vi "LSMcontroller_v64_updatedwaveformhandling.vi"() -> ()   [LabVIEW 2015] (continued)
                                "frames recorded" <- w3245
                                n916 = Greater?(x=w3258, y=w3260) -> (0:w3259:bool)
                                n917 = Quotient & Remainder(x=w3246, y=w3245) -> (floor(x/y)=w3247:i32)  [unwired: 1 out]
                                n918 = Transpose 2D Array(2D array=w3255) -> (transposed array=w3249:u16[][])
                                n919 = Transpose 2D Array(2D array=w3253) -> (transposed array=w3254:sgl[][])
                                n920 = And(x=w3259, y=w3248) -> (x .and. y?=w3261:bool)
                                n921 = local write "img_CH2"(w3254) -> ()
                                n922 = local write "photons/frame"(w3247) -> ()
                                n923 = Array Max & Min(array=w3249) -> (max value=w3250:u16)  [unwired: 3 out]
                                n924 = To Single Precision Float(number=w3249) -> (single precision float=w3252:sgl[][])
                                n925 = case shown="True" w3261 {
                                tunnel: w3260 -> [_ w3265]
                                frame False {
                                }
                                frame True {
                                n926 = Quotient & Remainder(x=w3265, y=u32 2 ("min phot")) -> (floor(x/y)=w3264:u32)  [unwired: 1 out]
                                n927 = Max & Min(x=w3264, y=u32 5) -> (max(x,y)=w3263:u32)  [unwired: 1 out]
                                n928 = local write "min phot"(w3263) -> ()
                                }
                                }
                                n929 = To Double Precision Float(number=w3250) -> (double precision float=w3251:dbl)
                                n930 = local write "img_CH1"(w3252) -> ()
                                n931 = property on="img_CH1" class="IntGraph (strict)"("ZScale.Maximum"=w3251) -> ()  [unwired: 2 in, 2 out]
                                }
                                }
                                }
                                frame #4 {
                                w3269 = u16 1 items=["Stream to disk", "Post process", "real time process"] ("Ring")
                                n932 = local read "T3R Data processing"() -> (w3268:u16)
                                n933 = Equal?(x=w3268, y=w3269) -> (x = y?=w3267:bool)
                                n934 = case shown="False" w3267 {
                                frame False {
                                # "intensity"
                                n935 = local read "Current Average"() -> (w3274:sgl)
                                n936 = local read "image2list"() -> (w3270:u16)
                                n937 = local read "image1list"() -> (w3271:u16)
                                n938 = call "dattoimage.vi"("image2list"=w3270, "Current Average"=w3274, "image1list"=w3271) -> ("image 1 array out"=w3273:sgl[][])  [unwired: 1 out]
                                n939 = Transpose 2D Array(2D array=w3273) -> (transposed array=w3272:sgl[][])
                                n940 = local write "img_CH2"(w3272) -> ()
                                }
                                frame True {
                                }
                                }
                                }
                                }
                              }
                              frame Enabled {
                              }
                            }
                          }
                        }
                        n941 = local write "64bit disabled"(TRUE ("64bit disabled")) -> ()
                      }
                      frame #9 {
                        n942 = call "2pparameters.vi"("command"="get") -> ("params out"=w3277:T10)  [unwired: 1 in]
                        n943 = Unbundle By Name(w3277) -> ("auto OD"=w3276:bool)
                        n944 = case shown="True" w3276 {
                          frame False {
                          }
                          frame True {
                            n945 = call "configuration.vi"("command"="get") -> ("config out"=w3280:T11)  [unwired: 2 in, 1 out]
                            n946 = call "2pparameters.vi"("command"="get") -> ("params out"=w3283:T10)  [unwired: 1 in]
                            n947 = Unbundle By Name(w3280) -> ("image OD"=w3278:u16)
                            n948 = Unbundle By Name(w3283) -> ("ODfilt"=w3279:u16)
                            n949 = call "filterwheelcontrol_nothorlabslib.vi"("Current OD filt"=w3278, "New ODfilt"=w3279) -> ()  [unwired: 1 in]
                          }
                        }
                        n950 = call "reset AO_DO_v3.vi"() -> ()  [unwired: 12 in]
                      }
                      frame #10 {
                        n951 = stacked-sequence {
                          tunnel: w3297 -> [w3300 _ _ _ _ _]
                          tunnel: w3296 -> [w3299 _ _ _ _ _]
                          tunnel: w3295 -> [w3298 _ _ _ _ _]
                          tunnel: w3294 -> [_ w3349 _ _ _ _]
                          tunnel: w3293 -> [_ w3348 w3403 w3500 _ _]
                          tunnel: w3292 -> [_ w3347 w3402 w3499 _ _]
                          tunnel: w3291 -> [_ _ w3401 _ _ _]
                          tunnel: w3290 -> [_ _ w3400 _ _ _]
                          tunnel: w3289 -> [_ _ _ w3498 _ _]
                          tunnel: w3288 -> [_ _ _ w3497 _ _]
                          tunnel: w3287 -> [_ _ w3398 _ _ _]
                          tunnel: w3286 -> [_ _ w3397 _ _ _]
                          tunnel: w3285 -> [_ _ _ w3495 _ _]
                          tunnel: w3284 -> [_ _ _ w3494 _ _]
                          frame #0 {
                            n952 = case shown="False" w3300 {
                              tunnel: w3299 -> [_ w3322]
                              tunnel: w3298 -> [_ w3321]
                              frame True {
                                n953 = stacked-sequence {
                                seq-local: [w3301 _ _] -> [_ w3313 w3318]
                                frame #0 {
                                n954 = call "configuration.vi"("command"="get") -> ("config out"=w3307:T11)  [unwired: 2 in, 1 out]
                                n955 = Unbundle By Name(w3307) -> ("Voltage to Xgalvo"=w3304:i32)
                                n956 = call "2pparameters.vi"("command"="get") -> ("params out"=w3305:T10)  [unwired: 1 in]
                                n957 = in-place {
                                in-place-border: w3304 -> [w3312]
                                in-place-border: [w3309] -> w3301
                                n958 = in-place-cluster #9(w3305) -> ("aAO"=w3311:u32[])
                                n959 = call "remove channel from active arrayv2.vi"("line array in"=w3311, "line to remove"=w3312) -> ("line array out"=w3310:u32[], "index"=w3309:i32)  [unwired: 1 out]
                                n960 = in-place-cluster #9("aAO"=w3310) -> (w3302:T10)
                                }
                                n961 = call "2pparameters.vi"("Params in"=w3302, "command"="set") -> ()  [unwired: 1 out]
                                }
                                frame #1 {
                                n962 = call "waveformparamsv2.vi"("command"="rem AO", "index"=w3313) -> ()  [unwired: 3 in, 3 out]
                                }
                                frame #2 {
                                n963 = call "waveformsAObuffer.vi"("command"="get") -> ("AO wf out"=w3319:waveform(dbl)[])  [unwired: 1 in]
                                n964 = Delete From Array(array=w3319, length=1, index=w3318) -> (array with subset deleted=w3315:waveform(dbl)[])  [unwired: 1 out]
                                n965 = call "waveformsAObuffer.vi"("AO wf in"=w3315, "command"="set") -> ()  [unwired: 1 out]
                                }
                                }
                              }
                              frame False {
                                n966 = stacked-sequence {
                                seq-local: [w3323 _ _] -> [_ w3331 w3342]
                                tunnel: w3322 -> [_ w3330 _]
                                tunnel: w3321 -> [_ _ w3341]
                                frame #0 {
                                n967 = call "configuration.vi"("command"="get") -> ("config out"=w3328:T11)  [unwired: 2 in, 1 out]
                                n968 = Unbundle By Name(w3328) -> ("Voltage to Xgalvo"=w3324:i32)
                                n969 = call "2pparameters.vi"("command"="get") -> ("params out"=w3327:T10)  [unwired: 1 in]
                                n970 = Unbundle By Name(w3327) -> ("aAO"=w3325:u32[])
                                n971 = Search 1D Array(1D array=w3325, element=w3324) -> (index of element=w3323:i32)  [unwired: 1 in]
                                }
                                frame #1 {
                                n972 = call "waveformparamsv2.vi"("command"="get") -> ("Params out"=w3334:T14)  [unwired: 4 in, 2 out]
                                n973 = in-place {
                                in-place-border: w3331 -> [w3338]
                                in-place-border: w3330 -> [w3337]
                                n974 = in-place-cluster #10(w3334) -> ("AO parameters"=w3339:T15)
                                n975 = in-place {
                                in-place-border: w3337 -> [w3340]
                                n976 = in-place-array #11(w3339, w3338) -> ()  [unwired: 1 out]
                                n977 = in-place-array #11(w3340) -> (w3336:T15)  [unwired: 1 out]
                                }
                                n978 = in-place-cluster #10("AO parameters"=w3336) -> (w3332:T14)
                                }
                                n979 = call "waveformparamsv2.vi"("command"="set", "Params in"=w3332) -> ()  [unwired: 3 in, 3 out]
                                }
                                frame #2 {
                                n980 = call "waveformsAObuffer.vi"("command"="get") -> ("AO wf out"=w3345:waveform(dbl)[])  [unwired: 1 in]
                                n981 = Replace Array Subset(array=w3345, new element=w3341, index=w3342) -> (w3343:waveform(dbl)[])
                                n982 = call "waveformsAObuffer.vi"("AO wf in"=w3343, "command"="set") -> ()  [unwired: 1 out]
                                }
                                }
                              }
                            }
                          }
                          frame #1 {
                            n983 = case shown="True" w3349 {
                              tunnel: w3348 -> [_ w3371]
                              tunnel: w3347 -> [_ w3370]
                              frame True {
                                n984 = stacked-sequence {
                                seq-local: [w3350 _ _] -> [_ w3362 w3367]
                                frame #0 {
                                n985 = call "configuration.vi"("command"="get") -> ("config out"=w3356:T11)  [unwired: 2 in, 1 out]
                                n986 = Unbundle By Name(w3356) -> ("Voltage to Ygalvo"=w3353:i32)
                                n987 = call "2pparameters.vi"("command"="get") -> ("params out"=w3354:T10)  [unwired: 1 in]
                                n988 = in-place {
                                in-place-border: w3353 -> [w3361]
                                in-place-border: [w3358] -> w3350
                                n989 = in-place-cluster #12(w3354) -> ("aAO"=w3360:u32[])
                                n990 = call "remove channel from active arrayv2.vi"("line array in"=w3360, "line to remove"=w3361) -> ("line array out"=w3359:u32[], "index"=w3358:i32)  [unwired: 1 out]
                                n991 = in-place-cluster #12("aAO"=w3359) -> (w3351:T10)
                                }
                                n992 = call "2pparameters.vi"("Params in"=w3351, "command"="set") -> ()  [unwired: 1 out]
                                }
                                frame #1 {
                                n993 = call "waveformparamsv2.vi"("command"="rem AO", "index"=w3362) -> ()  [unwired: 3 in, 3 out]
                                }
                                frame #2 {
                                n994 = call "waveformsAObuffer.vi"("command"="get") -> ("AO wf out"=w3368:waveform(dbl)[])  [unwired: 1 in]
                                n995 = Delete From Array(array=w3368, length=1, index=w3367) -> (array with subset deleted=w3364:waveform(dbl)[])  [unwired: 1 out]
                                n996 = call "waveformsAObuffer.vi"("AO wf in"=w3364, "command"="set") -> ()  [unwired: 1 out]
                                }
                                }
                              }
                              frame False {
                                n997 = stacked-sequence {
                                seq-local: [w3372 _ _] -> [_ w3380 w3391]
                                tunnel: w3371 -> [_ w3379 _]
                                tunnel: w3370 -> [_ _ w3390]
                                frame #0 {
                                n998 = call "configuration.vi"("command"="get") -> ("config out"=w3377:T11)  [unwired: 2 in, 1 out]
                                n999 = Unbundle By Name(w3377) -> ("Voltage to Ygalvo"=w3373:i32)
                                n1000 = call "2pparameters.vi"("command"="get") -> ("params out"=w3376:T10)  [unwired: 1 in]
                                n1001 = Unbundle By Name(w3376) -> ("aAO"=w3374:u32[])
                                n1002 = Search 1D Array(1D array=w3374, element=w3373) -> (index of element=w3372:i32)  [unwired: 1 in]
                                }
                                frame #1 {
                                n1003 = call "waveformparamsv2.vi"("command"="get") -> ("Params out"=w3383:T14)  [unwired: 4 in, 2 out]
                                n1004 = in-place {
                                in-place-border: w3380 -> [w3387]
                                in-place-border: w3379 -> [w3386]
                                n1005 = in-place-cluster #13(w3383) -> ("AO parameters"=w3388:T15)
                                n1006 = in-place {
                                in-place-border: w3386 -> [w3389]
                                n1007 = in-place-array #14(w3388, w3387) -> ()  [unwired: 1 out]
                                n1008 = in-place-array #14(w3389) -> (w3385:T15)  [unwired: 1 out]
                                }
                                n1009 = in-place-cluster #13("AO parameters"=w3385) -> (w3381:T14)
                                }
                                n1010 = call "waveformparamsv2.vi"("command"="set", "Params in"=w3381) -> ()  [unwired: 3 in, 3 out]
                                }
                                frame #2 {
                                n1011 = call "waveformsAObuffer.vi"("command"="get") -> ("AO wf out"=w3394:waveform(dbl)[])  [unwired: 1 in]
                                n1012 = Replace Array Subset(array=w3394, new element=w3390, index=w3391) -> (w3392:waveform(dbl)[])
                                n1013 = call "waveformsAObuffer.vi"("AO wf in"=w3392, "command"="set") -> ()  [unwired: 1 out]
                                }
                                }
                              }
                            }
                          }
                          frame #2 {
                            n1014 = Build Array(w3398, w3397) -> (w3396:bool[])
                            n1015 = Boolean Array To Number(Boolean array=w3396) -> (number=w3399:u32)
                            n1016 = case shown="0" w3399 {
                              tunnel: w3403 -> [_ _ w3446]
                              tunnel: w3402 -> [_ _ w3445]
                              tunnel: w3401 -> [_ w3425 w3443]
                              tunnel: w3400 -> [_ w3424 w3444]
                              frame 1, Default {
                                n1017 = stacked-sequence {
                                seq-local: [w3404 _ _] -> [_ w3416 w3421]
                                frame #0 {
                                n1018 = call "configuration.vi"("command"="get") -> ("config out"=w3410:T11)  [unwired: 2 in, 1 out]
                                n1019 = Unbundle By Name(w3410) -> ("2P shutter"=w3407:i32)
                                n1020 = call "2pparameters.vi"("command"="get") -> ("params out"=w3408:T10)  [unwired: 1 in]
                                n1021 = in-place {
                                in-place-border: w3407 -> [w3415]
                                in-place-border: [w3412] -> w3404
                                n1022 = in-place-cluster #15(w3408) -> ("aDO"=w3414:u32[])
                                n1023 = call "remove channel from active arrayv2.vi"("line array in"=w3414, "line to remove"=w3415) -> ("line array out"=w3413:u32[], "index"=w3412:i32)  [unwired: 1 out]
                                n1024 = in-place-cluster #15("aDO"=w3413) -> (w3405:T10)
                                }
                                n1025 = call "2pparameters.vi"("Params in"=w3405, "command"="set") -> ()  [unwired: 1 out]
                                }
                                frame #1 {
                                n1026 = call "waveformparamsv2.vi"("command"="rem DO", "index"=w3416) -> ()  [unwired: 3 in, 3 out]
                                }
                                frame #2 {
                                n1027 = call "waveformsDObuffer.vi"("command"="get") -> ("DO wf out"=w3422:digitalwaveform[])  [unwired: 1 in]
                                n1028 = Delete From Array(array=w3422, length=1, index=w3421) -> (array with subset deleted=w3418:digitalwaveform[])  [unwired: 1 out]
                                n1029 = call "waveformsDObuffer.vi"("DO wf in"=w3418, "command"="set") -> ()  [unwired: 1 out]
                                }
                                }
                              }
                              frame 2 {
                                n1030 = stacked-sequence {
                                tunnel: w3425 -> [_ w3436 _]
                                tunnel: w3424 -> [_ _ w3440]
                                frame #0 {
                                n1031 = call "configuration.vi"("command"="get") -> ("config out"=w3427:T11)  [unwired: 2 in, 1 out]
                                n1032 = call "2pparameters.vi"("command"="get") -> ("params out"=w3431:T10)  [unwired: 1 in]
                                n1033 = Unbundle By Name(w3427) -> ("2P shutter"=w3426:i32)
                                n1034 = in-place {
                                in-place-border: w3426 -> [w3435]
                                n1035 = in-place-cluster #16(w3431) -> ("aDO"=w3434:u32[])
                                n1036 = call "add channel to active arrayv2.vi"("line array in"=w3434, "line to add"=w3435) -> ("line array out"=w3433:u32[])  [unwired: 2 out]
                                n1037 = in-place-cluster #16("aDO"=w3433) -> (w3429:T10)
                                }
                                n1038 = call "2pparameters.vi"("Params in"=w3429, "command"="set") -> ()  [unwired: 1 out]
                                }
                                frame #1 {
                                n1039 = call "waveformparamsv2.vi"("command"="add DO", "add DO"=w3436) -> ()  [unwired: 3 in, 3 out]
                                }
                                frame #2 {
                                n1040 = call "waveformsDObuffer.vi"("command"="get") -> ("DO wf out"=w3441:digitalwaveform[])  [unwired: 1 in]
                                n1041 = Build Array (concatenate)(w3441, w3440) -> (w3439:digitalwaveform[])
                                n1042 = call "waveformsDObuffer.vi"("DO wf in"=w3439, "command"="set") -> ()  [unwired: 1 out]
                                }
                                }
                              }
                              frame 0 {
                                n1043 = stacked-sequence {
                                seq-local: [w3447 _ _] -> [_ w3455 w3477]
                                tunnel: w3446 -> [_ _ _]
                                tunnel: w3445 -> [_ _ _]
                                tunnel: w3444 -> [_ _ w3476]
                                tunnel: w3443 -> [_ w3454 _]
                                frame #0 {
                                n1044 = call "configuration.vi"("command"="get") -> ("config out"=w3452:T11)  [unwired: 2 in, 1 out]
                                n1045 = call "2pparameters.vi"("command"="get") -> ("params out"=w3451:T10)  [unwired: 1 in]
                                n1046 = Unbundle By Name(w3452) -> ("2P shutter"=w3448:i32)
                                n1047 = Unbundle By Name(w3451) -> ("aDO"=w3449:u32[])
                                n1048 = Search 1D Array(1D array=w3449, element=w3448) -> (index of element=w3447:i32)  [unwired: 1 in]
                                }
                                frame #1 {
                                n1049 = call "2pparameters.vi"("command"="get") -> ("params out"=w3458:T10)  [unwired: 1 in]
                                n1050 = Unbundle By Name(w3458) -> ("wavdet"=w3456:bool, "autoshutter"=w3457:bool)
                                n1051 = case shown="True" w3457 {
                                tunnel: w3455 -> [_ w3462]
                                tunnel: w3456 -> [_ w3461]
                                tunnel: w3454 -> [_ w3460]
                                frame False {
                                }
                                frame True {
                                n1052 = case shown="False" w3461 {
                                tunnel: w3462 -> [w3466 _]
                                tunnel: w3460 -> [w3464 _]
                                frame False {
                                n1053 = Index Array(array=w3464, index=0) -> (element=w3463:T18)
                                n1054 = call "waveformparamsv2.vi"("command"="get") -> ("Params out"=w3469:T14)  [unwired: 4 in, 2 out]
                                n1055 = in-place {
                                in-place-border: w3466 -> [w3473]
                                in-place-border: w3463 -> [w3471]
                                n1056 = in-place-cluster #17(w3469) -> ("DO parameters"=w3474:T17)
                                n1057 = in-place {
                                in-place-border: w3471 -> [w3475]
                                n1058 = in-place-array #18(w3474, w3473) -> ()  [unwired: 1 out]
                                n1059 = in-place-array #18(w3475) -> (w3472:T17)  [unwired: 1 out]
                                }
                                n1060 = in-place-cluster #17("DO parameters"=w3472) -> (w3467:T14)
                                }
                                n1061 = call "waveformparamsv2.vi"("command"="set", "Params in"=w3467) -> ()  [unwired: 3 in, 3 out]
                                }
                                frame True {
                                }
                                }
                                }
                                }
                                }
                                frame #2 {
                                n1062 = call "2pparameters.vi"("command"="get") -> ("params out"=w3480:T10)  [unwired: 1 in]
                                n1063 = Unbundle By Name(w3480) -> ("wavdet"=w3478:bool, "autoshutter"=w3479:bool)
                                n1064 = case shown="True" w3479 {
                                tunnel: w3477 -> [_ w3484]
                                tunnel: w3478 -> [_ w3483]
                                tunnel: w3476 -> [_ w3482]
                                frame False {
                                }
                                frame True {
                                n1065 = case shown="False" w3483 {
                                tunnel: w3484 -> [w3488 _]
                                tunnel: w3482 -> [w3487 _]
                                frame False {
                                n1066 = Index Array(array=w3487, index=0) -> (element=w3485:digitalwaveform)
                                n1067 = call "waveformsDObuffer.vi"("command"="get") -> ("DO wf out"=w3490:digitalwaveform[])  [unwired: 1 in]
                                n1068 = Replace Array Subset(array=w3490, new element=w3485, index=w3488) -> (w3492:digitalwaveform[])
                                n1069 = call "waveformsDObuffer.vi"("DO wf in"=w3492, "command"="set") -> ()  [unwired: 1 out]
                                }
                                frame True {
                                }
                                }
                                }
                                }
                                }
                                }
                              }
                            }
                          }
                          frame #3 {
                            n1070 = Build Array(w3495, w3494) -> (w3496:bool[])
                            n1071 = Boolean Array To Number(Boolean array=w3496) -> (number=w3493:u32)
                            n1072 = case shown="0" w3493 {
                              tunnel: w3500 -> [_ _ w3543]
                              tunnel: w3499 -> [_ _ w3542]
                              tunnel: w3498 -> [_ w3522 w3540]
                              tunnel: w3497 -> [_ w3521 w3541]
                              frame 1, Default {
                                n1073 = stacked-sequence {
                                seq-local: [w3501 _ _] -> [_ w3513 w3518]
                                frame #0 {
                                n1074 = call "configuration.vi"("command"="get") -> ("config out"=w3507:T11)  [unwired: 2 in, 1 out]
                                n1075 = Unbundle By Name(w3507) -> ("LT timestamp"=w3504:u32)
                                n1076 = call "2pparameters.vi"("command"="get") -> ("params out"=w3505:T10)  [unwired: 1 in]
                                n1077 = in-place {
                                in-place-border: w3504 -> [w3512]
                                in-place-border: [w3509] -> w3501
                                n1078 = in-place-cluster #19(w3505) -> ("aDO"=w3511:u32[])
                                n1079 = call "remove channel from active arrayv2.vi"("line array in"=w3511, "line to remove"=w3512) -> ("line array out"=w3510:u32[], "index"=w3509:i32)  [unwired: 1 out]
                                n1080 = in-place-cluster #19("aDO"=w3510) -> (w3502:T10)
                                }
                                n1081 = call "2pparameters.vi"("Params in"=w3502, "command"="set") -> ()  [unwired: 1 out]
                                }
                                frame #1 {
                                n1082 = call "waveformparamsv2.vi"("command"="rem DO", "index"=w3513) -> ()  [unwired: 3 in, 3 out]
                                }
                                frame #2 {
                                n1083 = call "waveformsDObuffer.vi"("command"="get") -> ("DO wf out"=w3519:digitalwaveform[])  [unwired: 1 in]
                                n1084 = Delete From Array(array=w3519, length=1, index=w3518) -> (array with subset deleted=w3515:digitalwaveform[])  [unwired: 1 out]
                                n1085 = call "waveformsDObuffer.vi"("DO wf in"=w3515, "command"="set") -> ()  [unwired: 1 out]
                                }
                                }
                              }
                              frame 2 {
                                n1086 = stacked-sequence {
                                tunnel: w3522 -> [_ _ w3535]
                                tunnel: w3521 -> [_ w3533 _]
                                frame #0 {
                                n1087 = call "configuration.vi"("command"="get") -> ("config out"=w3524:T11)  [unwired: 2 in, 1 out]
                                n1088 = Unbundle By Name(w3524) -> ("LT timestamp"=w3523:u32)
                                n1089 = call "2pparameters.vi"("command"="get") -> ("params out"=w3528:T10)  [unwired: 1 in]
                                n1090 = in-place {
                                in-place-border: w3523 -> [w3532]
                                n1091 = in-place-cluster #20(w3528) -> ("aDO"=w3531:u32[])
                                n1092 = call "add channel to active arrayv2.vi"("line array in"=w3531, "line to add"=w3532) -> ("line array out"=w3530:u32[])  [unwired: 2 out]
                                n1093 = in-place-cluster #20("aDO"=w3530) -> (w3526:T10)
                                }
                                n1094 = call "2pparameters.vi"("Params in"=w3526, "command"="set") -> ()  [unwired: 1 out]
                                }
                                frame #1 {
                                n1095 = call "waveformparamsv2.vi"("command"="add DO", "add DO"=w3533) -> ()  [unwired: 3 in, 3 out]
                                }
                                frame #2 {
                                n1096 = call "waveformsDObuffer.vi"("command"="get") -> ("DO wf out"=w3538:digitalwaveform[])  [unwired: 1 in]
                                n1097 = Build Array (concatenate)(w3538, w3535) -> (w3537:digitalwaveform[])
                                n1098 = call "waveformsDObuffer.vi"("DO wf in"=w3537, "command"="set") -> ()  [unwired: 1 out]
                                }
                                }
                              }
                              frame 0 {
                                n1099 = stacked-sequence {
                                seq-local: [w3544 _ _] -> [_ w3554 w3571]
                                tunnel: w3543 -> [_ _ _]
                                tunnel: w3542 -> [_ _ _]
                                tunnel: w3541 -> [_ w3551 _]
                                tunnel: w3540 -> [_ _ w3570]
                                frame #0 {
                                n1100 = call "configuration.vi"("command"="get") -> ("config out"=w3549:T11)  [unwired: 2 in, 1 out]
                                n1101 = Unbundle By Name(w3549) -> ("LT timestamp"=w3545:u32)
                                n1102 = call "2pparameters.vi"("command"="get") -> ("params out"=w3548:T10)  [unwired: 1 in]
                                n1103 = Unbundle By Name(w3548) -> ("aDO"=w3546:u32[])
                                n1104 = Search 1D Array(1D array=w3546, element=w3545) -> (index of element=w3544:i32)  [unwired: 1 in]
                                }
                                frame #1 {
                                n1105 = local read "Measurement"() -> (w3553:T4)
                                n1106 = To Unsigned Long Integer(number=w3553) -> (unsigned 32bit integer=w3552:u32)
                                n1107 = case shown="5..7" w3552 {
                                tunnel: w3554 -> [_ w3558]
                                tunnel: w3551 -> [_ w3555]
                                frame 0..4, Default {
                                }
                                frame 5..7 {
                                n1108 = Index Array(array=w3555, index=0) -> (element=w3556:T18)
                                n1109 = call "waveformparamsv2.vi"("command"="get") -> ("Params out"=w3561:T14)  [unwired: 4 in, 2 out]
                                n1110 = in-place {
                                in-place-border: w3558 -> [w3565]
                                in-place-border: w3556 -> [w3563]
                                n1111 = in-place-cluster #21(w3561) -> ("DO parameters"=w3566:T17)
                                n1112 = in-place {
                                in-place-border: w3563 -> [w3567]
                                n1113 = in-place-array #22(w3566, w3565) -> ()  [unwired: 1 out]
                                n1114 = in-place-array #22(w3567) -> (w3564:T17)  [unwired: 1 out]
                                }
                                n1115 = in-place-cluster #21("DO parameters"=w3564) -> (w3559:T14)
                                }
                                n1116 = call "waveformparamsv2.vi"("command"="set", "Params in"=w3559) -> ()  [unwired: 3 in, 3 out]
                                }
                                }
                                }
                                frame #2 {
                                n1117 = local read "Measurement"() -> (w3569:T4)
                                n1118 = To Unsigned Long Integer(number=w3569) -> (unsigned 32bit integer=w3568:u32)
                                n1119 = case shown="5..7" w3568 {
                                tunnel: w3571 -> [_ w3575]
                                tunnel: w3570 -> [_ w3573]
                                frame 0..4, Default {
                                }
                                frame 5..7 {
                                n1120 = Index Array(array=w3573, index=0) -> (element=w3572:digitalwaveform)
                                n1121 = call "waveformsDObuffer.vi"("command"="get") -> ("DO wf out"=w3577:digitalwaveform[])  [unwired: 1 in]
                                n1122 = Replace Array Subset(array=w3577, new element=w3572, index=w3575) -> (w3579:digitalwaveform[])
                                n1123 = call "waveformsDObuffer.vi"("DO wf in"=w3579, "command"="set") -> ()  [unwired: 1 out]
                                }
                                }
                                }
                                }
                              }
                            }
                          }
                          frame #4 {
                            n1124 = call "Used AO lines.vi"() -> ("used AO names"=w3582:string[], "used AO lines"=w3580:tag[])  [unwired: 2 in]
                            n1125 = control-ref of="Analog Lines Plot"() -> (w3581:refnum<vi>)
                            n1126 = control-ref of="Digital Lines Plot"() -> (w3583:refnum<vi>)
                            n1127 = call "Used DO lines.vi"() -> ("used DO names"=w3584:string[], "used DO lines"=w3585:tag[])  [unwired: 2 in]
                            n1128 = local write "Analog Used Lines"(w3580) -> ()
                            n1129 = local write "Analog Used Names"(w3582) -> ()
                            n1130 = local write "Digital Used Lines"(w3585) -> ()
                            n1131 = local write "Digital Used Names"(w3584) -> ()
                            n1132 = call "prepDOWaveplot.vi"("DigitalGraph in"=w3583, "used DO names"=w3584) -> ()  [unwired: 1 in]
                            n1133 = call "prepAOWaveplot.vi"("WaveformGraph in"=w3581, "Analog Used Names"=w3582) -> ()  [unwired: 1 in]
                          }
                          frame #5 {
                            n1134 = local read "Meastab"() -> (w3600:enum32{"X-Y Image", "Linescan", "Timetrace"})
                            n1135 = property on="refwf" class="Ring (strict)"() -> ("RingText.Text"=w3597:string)  [unwired: 2 in, 2 out]
                            n1136 = case shown="\"Timetrace\"" w3600 {
                              tunnel: [w3602 w3603] -> w3601
                              frame "X-Y Image", Default {
                                n1137 = local read "Sampling rate"() -> (w3602:dbl)
                              }
                              frame "Timetrace" {
                                n1138 = local read "srateAODOtt"() -> (w3603:dbl)
                              }
                            }
                            n1139 = call "waveformsAObuffer.vi"("command"="get") -> ("AO wf out"=w3588:waveform(dbl)[])  [unwired: 1 in]
                            n1140 = local read "wavdet"() -> (w3598:bool)
                            n1141 = call "waveformsDObuffer.vi"("command"="get") -> ("DO wf out"=w3592:digitalwaveform[])  [unwired: 1 in]
                            n1142 = call "correctwaveformsizetemp.vi"("new sampling frequency (Hz)"=w3601, "start"=FALSE, "reference waveforms to"=w3597, "Analog waveforms in"=w3588, "stop"=TRUE, "Digital waveforms in"=w3592) -> ("analog wf out"=w3594:waveform(dbl)[], "Digital wf out"=w3596:digitalwaveform[], "measpoints"=w3599:i32)
                            n1143 = local write "Analog Lines Plot"(w3594) -> ()
                            n1144 = call "GetNumCamFramesv2.vi"("Digital Waveform Graph"=w3596) -> ("Numeric"=w3595:i32)  [unwired: 10 in]
                            n1145 = local write "Digital Lines Plot"(w3596) -> ()
                            n1146 = call "waveformsDObuffer.vi"("DO wf in"=w3596, "command"="set") -> ()  [unwired: 1 out]
                            n1147 = call "waveformsAObuffer.vi"("AO wf in"=w3594, "command"="set") -> ()  [unwired: 1 out]
                            n1148 = local write "Total Camera Frames"(w3595) -> ()
                            n1149 = case shown="True" w3598 {
                              tunnel: w3599 -> [_ w3604]
                              frame False {
                              }
                              frame True {
                                n1150 = local write "# of frames"(w3604) -> ()
                              }
                            }
                          }
                        }
                        n1151 = call "stoperaseCI.vi"() -> ()  [unwired: 12 in]
                        n1152 = call "stoperaseDO_img.vi"() -> ()  [unwired: 12 in]
                        n1153 = call "stoperaseAO_img.vi"() -> ()  [unwired: 12 in]
                        n1154 = call "stoperaseAI_img.vi"() -> ()  [unwired: 12 in]
                      }
                      frame #11 {
                        w3612 = FALSE ("Value (Signaling)")
                        n1155 = local read "save\ndata"() -> (w3605:bool)
                        n1156 = local read "save\ndata"() -> (w3606:bool)
                        n1157 = property on="Stop" class="Bool (strict)"("Visible"=FALSE, "DisabledEnum"=T7."Disabled" ("Disabled")) -> ()  [unwired: 2 in, 2 out]
                        n1158 = case shown="True" w3605 {
                          frame False {
                          }
                          frame True {
                            n1159 = call "closetiffs.vi"() -> ()  [unwired: 12 in]
                          }
                        }
                        n1160 = case shown="True" w3606 {
                          tunnel: w3607 -> [_ w3613]
                          frame False {
                          }
                          frame True {
                            n1161 = local read "filename prefix"() -> (w3615:string)
                            n1162 = local read "data dir"() -> (w3614:path)
                            n1163 = call "savetimestamps.vi"("timestamp"=w3613, "filename prefix in"=w3615, "data dir in"=w3614) -> ()  [unwired: 1 in]
                            n1164 = call "saveparams.vi"("filename prefix in"=w3615, "data dir in"=w3614) -> ()  [unwired: 2 in]
                          }
                        }
                        n1165 = property on="Start" class="Bool (strict)"("Visible"=TRUE, "DisabledEnum"=T7."Enabled" ("Disabled")) -> ()  [unwired: 2 in, 2 out]
                        n1166 = property on="Start" class="Bool (strict)"("Val(Sgnl)"=w3612) -> ()  [unwired: 2 in, 2 out]
                        n1167 = property on="Stop" class="Bool (strict)"("Val(Sgnl)"=w3612) -> ()  [unwired: 2 in, 2 out]
                      }
                      frame #12 {
                        w3619 = T21 2 items=["no dialog", "OK message", "continue or stop message", "OK message + warnings", "continue/stop + warnings"] ("type of dialog (OK msg:1)")
                        n1168 = call "displayerrors.vi"() -> ("error IO"=w3618:errorcluster)
                        n1169 = call <vilib>:"General Error Handler.vi"("type of dialog (OK msg:1)"=w3619, "error in (no error)"=w3618) -> ("error out"=w3617:errorcluster)  [unwired: 9 in, 4 out]
                        n1170 = call <vilib>:"Clear Errors.vi"("error in (no error)"=w3617) -> ("error out"=w3616:errorcluster)  [unwired: 5 in, 1 out]
                        n1171 = call "seterrors.vi"("error IO"=w3616) -> ()
                      }
                    }
                  }
                  frame "X-Y-Z-t movie" {
                    n1172 = call "2pparameters.vi"("command"="get") -> ("params out"=w3622:T10)  [unwired: 1 in]
                    n1173 = Bundle By Name(cluster=w3622, "type"="X-Y-Z-t movie") -> (w3620:T10)
                    n1174 = call "2pparameters.vi"("Params in"=w3620, "command"="set") -> ()  [unwired: 1 out]
                  }
                  frame "linescan" {
                    n1175 = call "2pparameters.vi"("command"="get") -> ("params out"=w3627:T10)  [unwired: 1 in]
                    n1176 = Bundle By Name(cluster=w3627, "type"="linescan") -> (w3629:T10)
                    n1177 = call "2pparameters.vi"("Params in"=w3629, "command"="set") -> ()  [unwired: 1 out]
                  }
                  frame "Timetrace", "Lifetime (contour)" {
                    n1178 = local read "ttt"() -> (w3630:T3)
                    n1179 = case shown="\"Point\", \"Resonant Ellipse\", \"freeform contour\", \"Fill Ellipse\", Default" w3630 {
                      selector: w3630 -> [_ w3631]
                      frame "Line" {
                      }
                      frame "Point", "Resonant Ellipse", "freeform contour", "Fill Ellipse", Default {
                        n1180 = stacked-sequence {
                          seq-local: [w3647 _ _ _ _ _ _ _ _ _ _] -> [_ _ w4520 _ _ w4533 w4600 _ _ w4960 _]
                          seq-local: [w3646 _ _ _ _ _ _ _ _ _ _] -> [_ _ _ _ _ _ _ _ w4647 _ _]
                          seq-local: [w3645 _ _ _ _ _ _ _ _ _ _] -> [_ _ _ _ _ _ _ _ w4646 _ _]
                          seq-local: [w3644 _ _ _ _ _ _ _ _ _ _] -> [_ _ _ _ _ _ _ _ w4649 _ _]
                          seq-local: [w3643 _ _ _ _ _ _ _ _ _ _] -> [_ _ _ _ _ _ _ _ w4645 _ _]
                          seq-local: [w3642 _ _ _ _ _ _ _ _ _ _] -> [_ _ _ _ _ _ _ _ w4644 _ _]
                          seq-local: [w3641 _ _ _ _ _ _ _ _ _ _] -> [_ _ _ _ _ _ _ _ w4648 _ _]
                          seq-local: [w3640 _ _ _ _ _ _ _ _ _ _] -> [_ _ _ _ _ _ _ _ w4643 _ _]
                          seq-local: [w3639 _ _ _ _ _ _ _ _ _ _] -> [_ _ _ _ _ _ _ _ w4642 _ _]
                          seq-local: [w3638 _ _ _ _ _ _ _ _ _ _] -> [_ _ _ _ _ _ _ _ w4637 _ _]
                          seq-local: [w3637 _ _ _ _ _ _ _ _ _ _] -> [_ _ _ _ _ _ _ _ w4636 _ _]
                          seq-local: [w3636 _ _ _ _ _ _ _ _ _ _] -> [_ _ _ _ _ _ _ _ w4641 _ _]
                          seq-local: [w3635 _ _ _ _ _ _ _ _ _ _] -> [_ _ _ _ _ _ _ _ w4640 _ _]
                          seq-local: [w3634 _ _ _ _ _ _ _ _ _ _] -> [_ _ _ _ _ _ _ _ w4639 _ _]
                          seq-local: [w3633 _ _ _ _ _ _ _ _ _ _] -> [_ _ _ _ _ _ _ _ w4638 _ _]
                          tunnel: w3631 -> [w3632 _ _ _ _ _ _ _ _ _ _]
                          frame #0 {
                            n1181 = local read "save\ndata"() -> (w3648:bool)
                            n1182 = Get Date/Time In Seconds() -> (seconds since 1Jan1904=w3649:timestamp)
                            n1183 = case shown="False" w3648 {
                              tunnel: w3649 -> [w3650 w3652]
                              tunnel: [w3650 w3651] -> w3647
                              frame False {
                              }
                              frame True {
                                n1184 = call "createdatafolder.vi"("timestamp in"=w3652) -> ("current data path"=w3653:path, "timestamp out"=w3651:timestamp)
                                n1185 = local write "data dir"(w3653) -> ()
                              }
                            }
                            n1186 = stacked-sequence {
                              tunnel: w3647 -> [w3659 _ _ _ _ _ _ _ _]
                              tunnel: [_ _ _ _ _ _ w3825 _ _] -> w3646
                              tunnel: [_ _ _ _ _ _ w3824 _ _] -> w3645
                              tunnel: [_ _ _ _ _ _ w3823 _ _] -> w3644
                              tunnel: [_ _ _ _ _ _ w3822 _ _] -> w3643
                              tunnel: [_ _ _ _ _ _ w3821 _ _] -> w3642
                              tunnel: [_ _ _ _ _ _ w3820 _ _] -> w3641
                              tunnel: [_ _ _ _ _ _ w3819 _ _] -> w3640
                              tunnel: [_ _ _ _ _ _ w3818 _ _] -> w3639
                              tunnel: [_ _ _ _ _ _ w3817 _ _] -> w3638
                              tunnel: [_ _ _ _ _ _ w3816 _ _] -> w3637
                              tunnel: [_ _ _ _ _ _ w3815 _ _] -> w3636
                              tunnel: [_ _ _ _ _ _ w3814 _ _] -> w3635
                              tunnel: [_ _ _ _ _ _ w3813 _ _] -> w3634
                              tunnel: [_ _ _ _ _ _ w3812 _ _] -> w3633
                              tunnel: w3632 -> [_ _ w3697 _ w3756 _ _ _ _]
                              frame #0 {
                                n1187 = local write "graphtab"(T5."timetrace" ("graphtab")) -> ()
                                n1188 = local read "AI channels"() -> (w3663:i32[])
                                n1189 = local read "CI channels"() -> (w3664:i32[])
                                n1190 = property on="Stop" class="Bool (strict)"("Visible"=TRUE, "DisabledEnum"=T7."Enabled" ("Disabled")) -> ()  [unwired: 2 in, 2 out]
                                n1191 = property on="Start" class="Bool (strict)"("Visible"=FALSE, "DisabledEnum"=T7."Disabled and Grayed Out" ("Disabled")) -> ()  [unwired: 2 in, 2 out]
                                n1192 = Format Date/Time String(time format string (%c)="%Y%m%d", seconds (now)=w3659) -> (date/time string=w3658:string)  [unwired: 1 in]
                                n1193 = Format Date/Time String(time format string (%c)="%H%M%S", seconds (now)=w3659) -> (date/time string=w3657:string)  [unwired: 1 in]
                                n1194 = call "2pparameters.vi"("command"="get") -> ("params out"=w3666:T10)  [unwired: 1 in]
                                n1195 = Bundle By Name(cluster=w3666, "aAI"=w3663, "aCI"=w3664, "type"="Timetrace", "date"=w3658, "time"=w3657) -> (w3665:T10)
                                n1196 = call "X-array-databuffer.vi"("command"=enum16{"get", "set", "clear", "append"}."clear") -> ()  [unwired: 3 in, 2 out]
                                n1197 = call "Y-array-databuffer.vi"("command"=enum16{"get", "set", "clear", "append"}."clear") -> ()  [unwired: 3 in, 2 out]
                                n1198 = call "2pparameters.vi"("Params in"=w3665, "command"="set") -> ()  [unwired: 1 out]
                                n1199 = call "CH1-1D-temp.vi"("command"=enum16{"get", "set", "clear", "append"}."clear") -> ()  [unwired: 3 in, 2 out]
                                n1200 = call "CH2-1D-temp.vi"("command"=enum16{"get", "set", "clear", "append"}."clear") -> ()  [unwired: 3 in, 2 out]
                                n1201 = call "allAI-temp.vi"("command"=enum16{"get", "set", "clear", "append"}."clear") -> ()  [unwired: 3 in, 2 out]
                              }
                              frame #1 {
                                n1202 = call "configuration.vi"("command"="get") -> ("config out"=w3683:T11)  [unwired: 2 in, 1 out]
                                n1203 = Unbundle By Name(w3683) -> ("CI names"=w3684:string[], "AI names"=w3685:string[])
                                n1204 = call "2pparameters.vi"("command"="get") -> ("params out"=w3679:T10)  [unwired: 1 in]
                                n1205 = Unbundle By Name(w3679) -> ("aCI"=w3680:i32[], "aAI"=w3681:i32[])
                                n1206 = for {
                                tunnel: w3680 -> [w3695] mode=indexing
                                tunnel: w3684 -> [w3696]
                                tunnel: [w3694] -> w3686 mode=indexing
                                n1207 = Index Array(array=w3696, index=w3695) -> (element=w3694:string)
                                }
                                n1208 = for {
                                tunnel: w3681 -> [w3692] mode=indexing
                                tunnel: w3685 -> [w3693]
                                tunnel: [w3691] -> w3687 mode=indexing
                                n1209 = Index Array(array=w3693, index=w3692) -> (element=w3691:string)
                                }
                                n1210 = Build Array (concatenate)(w3686, w3687) -> (w3677:string[])
                                n1211 = for {
                                tunnel: w3677 -> [w3689] mode=indexing
                                tunnel: [w3688] -> w3676 mode=indexing
                                i -> [w3690]
                                n1212 = Bundle("String"=w3689, w3690) -> (w3688:cluster{"String":string, i32})  [unwired: 1 in]
                                }
                                n1213 = property on="graph1list" class="Ring (strict)"("StringsAndValues[]"=w3676) -> ()  [unwired: 2 in, 2 out]
                                n1214 = property on="graph2list" class="Ring (strict)"("StringsAndValues[]"=w3676) -> ()  [unwired: 2 in, 2 out]
                              }
                              frame #2 {
                                n1215 = call "2pparameters.vi"("command"="get") -> ("params out"=w3700:T10)  [unwired: 1 in]
                                n1216 = Unbundle By Name(w3700) -> ("auto OD"=w3698:bool, "autoshutter"=w3701:bool)
                                n1217 = case shown="True" w3698 {
                                tunnel: w3697 -> [_ w3702]
                                frame False {
                                }
                                frame True {
                                n1218 = case shown="\"Point\"" w3702 {
                                frame "Point" {
                                n1219 = call "configuration.vi"("command"="get") -> ("config out"=w3705:T11)  [unwired: 2 in, 1 out]
                                n1220 = Unbundle By Name(w3705) -> ("point OD"=w3706:u16)
                                n1221 = local read "ODfilt"() -> (w3703:u16)
                                n1222 = call "filterwheelcontrol_nothorlabslib.vi"("Current OD filt"=w3703, "New ODfilt"=w3706) -> ()  [unwired: 1 in]
                                }
                                frame "Resonant Ellipse", Default {
                                n1223 = call "configuration.vi"("command"="get") -> ("config out"=w3709:T11)  [unwired: 2 in, 1 out]
                                n1224 = Unbundle By Name(w3709) -> ("contour OD"=w3710:u16)
                                n1225 = local read "ODfilt"() -> (w3707:u16)
                                n1226 = call "filterwheelcontrol_nothorlabslib.vi"("Current OD filt"=w3707, "New ODfilt"=w3710) -> ()  [unwired: 1 in]
                                }
                                }
                                }
                                }
                                n1227 = case shown="True" w3701 {
                                frame False {
                                }
                                frame True {
                                n1228 = call "shuttercontrol.vi"("command"="close") -> ()  [unwired: 1 in, 1 out]
                                }
                                }
                              }
                              frame #3 {
                                n1229 = local read "Vy-min draw"() -> (w3719:dbl)
                                n1230 = local read "Vy-max draw"() -> (w3718:dbl)
                                n1231 = local read "Vx-min draw"() -> (w3721:dbl)
                                n1232 = local read "Vx-max draw"() -> (w3720:dbl)
                                n1233 = local read "xpixels ref"() -> (w3717:i32)
                                n1234 = local read "ypixels ref"() -> (w3716:i32)
                                n1235 = local read "ROI Type"() -> (w3715:u16)
                                n1236 = local read "srateAODOtt"() -> (w3738:dbl)
                                n1237 = local read "# of frames"() -> (w3743:i32)
                                n1238 = local read "refreshtime"() -> (w3735:dbl)
                                n1239 = local read "Pel"() -> (w3714:dbl)
                                n1240 = local read "bin"() -> (w3741:dbl)
                                n1241 = local read "Override AI buffer"() -> (w3712:bool)
                                n1242 = local read "finite samples"() -> (w3750:bool)
                                n1243 = local read "srateAODOtt"() -> (w3737:dbl)
                                n1244 = local read "srateAODOtt"() -> (w3744:dbl)
                                n1245 = local read "continuous"() -> (w3749:bool)
                                n1246 = local read "Angle ref"() -> (w3722:dbl)
                                n1247 = local read "wavdet"() -> (w3751:bool)
                                n1248 = local read "Vx-ref"() -> (w3746:dbl)
                                n1249 = local read "Vy-ref"() -> (w3748:dbl)
                                n1250 = local read "avpp"() -> (w3747:i32)
                                n1251 = call "tt_timeandsamples.vi"("bin"=w3741, "refreshtime"=w3735, "srateAODOtt"=w3738, "tot#ofsamples"=w3743) -> ("refreshrate"=w3739:dbl, "refreshbuffer"=w3740:i32, "timetracecycles"=w3745:i32)  [unwired: 5 in]
                                n1252 = local read "bin"() -> (w3742:dbl)
                                n1253 = call "2pparameters.vi"("command"="get") -> ("params out"=w3754:T10)  [unwired: 1 in]
                                n1254 = Bundle By Name(cluster=w3754, "Drawing Mode"=w3715, "measpoints"=w3743, "tt_cycles"=w3745, "refreshbuffer"=w3740, "refreshrate"=w3739, "Vx-ref"=w3746, "Vy-ref"=w3748, "srate"=w3737, "finite"=w3750, "cont"=w3749, "wavdet"=w3751, "avpp"=w3747, "srateAODO"=w3744, "bufferAI"=w3740, "bin"=w3742, "Angle Img"=w3722, "Vxminref"=w3721, "Vxmaxref"=w3720, "Vyminref"=w3719, "Vymaxref"=w3718, "Xpixels Img"=w3717, "Ypixels Img"=w3716, "Pel"=w3714, "Vz-reset"=0.0, "AIoverride"=w3712) -> (w3752:T10)
                                n1255 = Reciprocal(x=w3739) -> (1/x=w3736:dbl)
                                n1256 = local write "refreshtime"(w3736) -> ()
                                n1257 = call "2pparameters.vi"("Params in"=w3752, "command"="set") -> ()  [unwired: 1 out]
                                n1258 = local read "Voltage Clamp"() -> (w3729:bool)
                                n1259 = local read "Current Clamp"() -> (w3730:bool)
                                n1260 = local read "Vholding (mV)"() -> (w3724:sgl)
                                n1261 = local read "CC_ICgain"() -> (w3728:dbl)
                                n1262 = local read "OCgain"() -> (w3725:sgl)
                                n1263 = local read "holdon"() -> (w3723:bool)
                                n1264 = call "patchparameters.vi"("command"="get") -> ("Params out"=w3732:T13)  [unwired: 1 in]
                                n1265 = Bundle By Name(cluster=w3732, "VC"=w3729, "CC"=w3730, "CC_icg (pA/mv)"=w3728, "VC_icg (mV/mV)"=10.0, "OCG (mV/pA)"=w3725, "OVG (mV/mV)"=0.1, "Vhold (mV)"=w3724, "holdon"=w3723) -> (w3731:T13)
                                n1266 = call "patchparameters.vi"("Params in"=w3731, "command"="set") -> ()  [unwired: 1 out]
                              }
                              frame #4 {
                                n1267 = case shown="\"Point\"" w3756 {
                                frame "Point" {
                                n1268 = call "2pparameters.vi"("command"="get") -> ("params out"=w3772:T10)  [unwired: 1 in]
                                n1269 = Unbundle By Name(w3772) -> ("Pel"=w3761:sgl, "Vx-min Img"=w3774:dbl, "VX-max Img"=w3773:dbl, "Vy-min Img"=w3776:dbl, "Vy-max Img"=w3775:dbl, "Angle Img"=w3777:dbl, "Vx-ref"=w3770:dbl, "Vy-ref"=w3769:dbl)
                                n1270 = script code="Xic=(ximax+ximin)./2;\nYic=(yimax+yimin)./2;\nx=x-Xic;\ny=y-Yic;\nxout=x.*cos(pi/180.*phi)+y.*sin(pi./180.*phi)+Xic;\nyout=-x.*sin(pi./180.*phi)+y.*cos(pi./180.*phi)+Yic;"("ximax"=w3773, "ximin"=w3774, "yimax"=w3775, "yimin"=w3776, "phi"=w3777, "x"=w3770, "y"=w3769) -> ("xout"=w3763:dbl, "yout"=w3762:dbl)  [unwired: 1 in, 1 out]
                                n1271 = call "2pparameters.vi"("command"="get") -> ("params out"=w3765:T10)  [unwired: 1 in]
                                n1272 = Bundle By Name(cluster=w3765, "P"=0.0) -> (w3768:T10)
                                n1273 = Initialize Array(w3762, w3761) -> (w3759:dbl[])
                                n1274 = Initialize Array(w3763, w3761) -> (w3758:dbl[])
                                n1275 = call "2pparameters.vi"("Params in"=w3768, "command"="set") -> ()  [unwired: 1 out]
                                n1276 = call "X-array-databuffer.vi"("array in"=w3758, "command"=enum16{"get", "set", "clear", "append"}."set") -> ()  [unwired: 2 in, 2 out]
                                n1277 = call "Y-array-databuffer.vi"("array in"=w3759, "command"=enum16{"get", "set", "clear", "append"}."set") -> ()  [unwired: 2 in, 2 out]
                                }
                                frame "Resonant Ellipse", Default {
                                n1278 = call "2pparameters.vi"("command"="get") -> ("params out"=w3792:T10)  [unwired: 1 in]
                                n1279 = Unbundle By Name(w3792) -> ("srateAODO"=w3793:sgl, "Angle Img"=w3794:dbl, "Angle draw"=w3795:dbl, "Vxmaxref"=w3796:dbl, "Vxminref"=w3797:dbl, "Xpixels Img"=w3798:i32, "Ypixels Img"=w3799:i32, "Vymaxref"=w3800:dbl, "Vxminref"=w3801:dbl, "Drawing Mode"=w3802:u16, "Pel"=w3803:sgl)
                                n1280 = Add(x=w3794, y=w3795) -> (x+y=w3778:dbl)
                                n1281 = call "ROI-databuffer.vi"("command"=enum16{"get", "set", "clear", "append"}."get") -> ("array out"=w3786:cluster{"x":sgl, "y":sgl}[])  [unwired: 4 in]
                                n1282 = call "ScanningWaveform_v4.vi"("Vy-min"=w3801, "Vy-max"=w3800, "yPixels/tPixels"=w3799, "xPixels/rPixels"=w3798, "Vx-min"=w3797, "Vx-max"=w3796, "Drawing Mode"=w3802, "Angle"=w3778, "AOrate"=w3793, "Points"=w3786, "points in ellipse"=w3803) -> ("numPixels"=w3779:dbl, "Y-WaveArray"=w3780:dbl[], "P"=w3785:dbl, "X-WaveArray"=w3781:dbl[])  [unwired: 5 in]
                                n1283 = call "Y-array-databuffer.vi"("array in"=w3780, "command"=enum16{"get", "set", "clear", "append"}."set") -> ()  [unwired: 2 in, 2 out]
                                n1284 = call "X-array-databuffer.vi"("array in"=w3781, "command"=enum16{"get", "set", "clear", "append"}."set") -> ()  [unwired: 2 in, 2 out]
                                n1285 = call "2pparameters.vi"("command"="get") -> ("params out"=w3790:T10)  [unwired: 1 in]
                                n1286 = Bundle By Name(cluster=w3790, "P"=w3785, "sAOxy"=w3779, "Pel"=w3779) -> (w3782:T10)
                                n1287 = call "2pparameters.vi"("Params in"=w3782, "command"="set") -> ()  [unwired: 1 out]
                                }
                                }
                              }
                              frame #5 {
                                n1288 = call "X-array-databuffer.vi"("command"=enum16{"get", "set", "clear", "append"}."get") -> ("array out"=w3806:dbl[])  [unwired: 3 in, 1 out]
                                n1289 = call "Y-array-databuffer.vi"("command"=enum16{"get", "set", "clear", "append"}."get") -> ("array out"=w3809:dbl[])  [unwired: 3 in, 1 out]
                                n1290 = Index Array(array=w3806, index=0) -> (element=w3805:dbl)
                                n1291 = Index Array(array=w3809, index=0) -> (element=w3804:dbl)
                                n1292 = call "setposition.vi"("Vy"=w3804, "Vx"=w3805) -> ()  [unwired: 1 in]
                              }
                              frame #6 {
                                # "rem2Ps"
                                # "A2Ps"
                                # "Al"
                                # "Rl"
                                n1293 = stacked-sequence {
                                seq-local: [w3830 _ _ _ _ _ _ _ _ _ _] -> [_ w3942 _ w4003 _ w4089 _ _ _ _ _]
                                seq-local: [w3831 _ _ _ _ _ _ _ _ _ _] -> [_ w3943 w3953 _ w4058 _ _ _ _ _ _]
                                seq-local: [_ _ w3952 _ _ _ _ _ _ _ _] -> [_ _ _ _ w4052 _ _ _ _ _ _]
                                seq-local: [_ _ _ w4002 _ _ _ _ _ _ _] -> [_ _ _ _ _ w4088 _ _ _ _ _]
                                seq-local: [w3827 _ _ _ _ _ _ _ _ _ _] -> [_ w3939 _ _ _ _ _ _ w4274 w4342 _]
                                seq-local: [w3826 _ _ _ _ _ _ _ _ _ _] -> [_ w3938 _ _ _ _ _ _ w4275 w4343 _]
                                seq-local: [w3833 _ _ _ _ _ _ _ _ _ _] -> [_ _ _ _ _ _ w4127 _ w4273 w4341 _]
                                seq-local: [w3829 _ _ _ _ _ _ _ _ _ _] -> [_ w3937 _ _ _ _ w4126 w4194 _ _ _]
                                seq-local: [w3828 _ _ _ _ _ _ _ _ _ _] -> [_ w3936 _ _ _ _ w4125 w4193 _ _ _]
                                seq-local: [w3832 _ _ _ _ _ _ _ _ _ _] -> [_ _ _ _ _ _ w4124 w4192 _ _ _]
                                tunnel: [_ _ w3951 _ _ _ _ _ _ _ _] -> w3824
                                tunnel: [_ _ w3950 _ _ _ _ _ _ _ _] -> w3825
                                tunnel: [w3831 _ _ _ _ _ _ _ _ _ _] -> w3823
                                tunnel: [w3830 _ _ _ _ _ _ _ _ _ _] -> w3820
                                tunnel: [_ _ _ w4001 _ _ _ _ _ _ _] -> w3821
                                tunnel: [_ _ _ w4000 _ _ _ _ _ _ _] -> w3822
                                tunnel: [w3829 _ _ _ _ _ _ _ _ _ _] -> w3815
                                tunnel: [w3828 _ _ _ _ _ _ _ _ _ _] -> w3814
                                tunnel: [_ _ _ _ _ _ w4123 _ _ _ _] -> w3813
                                tunnel: [_ _ _ _ _ _ _ w4191 _ _ _] -> w3812
                                tunnel: [w3827 _ _ _ _ _ _ _ _ _ _] -> w3816
                                tunnel: [w3826 _ _ _ _ _ _ _ _ _ _] -> w3817
                                tunnel: [_ _ _ _ _ _ _ _ w4272 _ _] -> w3818
                                tunnel: [_ _ _ _ _ _ _ _ _ w4340 _] -> w3819
                                frame #0 {
                                # "for a next version, give ome thought to\nthe possibilit of intermittently updating the\nwaveforms. it will have to be a calculation\nbased on speed of CPU and program on the one hand\nand length of measurement on the other. but then it should be possible, in principle, to \nupdate the waveform on the fly and that way cut up a longer measurement in smaller parts."
                                n1294 = stacked-sequence {
                                tunnel: [w3834 _ _ _] -> w3831
                                tunnel: [_ w3846 _ _] -> w3830
                                tunnel: [_ _ _ w3903] -> w3826
                                tunnel: [_ _ _ w3902] -> w3827
                                tunnel: [_ _ _ w3901] -> w3833
                                tunnel: [_ _ w3861 _] -> w3829
                                tunnel: [_ _ w3860 _] -> w3828
                                tunnel: [_ _ w3859 _] -> w3832
                                frame #0 {
                                n1295 = call "configuration.vi"("command"="get") -> ("config out"=w3836:T11)  [unwired: 2 in, 1 out]
                                n1296 = Unbundle By Name(w3836) -> ("Voltage to Xgalvo"=w3835:i32)
                                n1297 = call "2pparameters.vi"("command"="get") -> ("params out"=w3840:T10)  [unwired: 1 in]
                                n1298 = in-place {
                                in-place-border: w3835 -> [w3845]
                                in-place-border: [w3842] -> w3834
                                n1299 = in-place-cluster #23(w3840) -> ("aAO"=w3844:u32[])
                                n1300 = call "add channel to active arrayv2.vi"("line array in"=w3844, "line to add"=w3845) -> ("line array out"=w3843:u32[], "addition"=w3842:bool)  [unwired: 1 out]
                                n1301 = in-place-cluster #23("aAO"=w3843) -> (w3838:T10)
                                }
                                n1302 = call "2pparameters.vi"("Params in"=w3838, "command"="set") -> ()  [unwired: 1 out]
                                }
                                frame #1 {
                                n1303 = call "configuration.vi"("command"="get") -> ("config out"=w3848:T11)  [unwired: 2 in, 1 out]
                                n1304 = Unbundle By Name(w3848) -> ("Voltage to Ygalvo"=w3847:i32)
                                n1305 = call "2pparameters.vi"("command"="get") -> ("params out"=w3852:T10)  [unwired: 1 in]
                                n1306 = in-place {
                                in-place-border: w3847 -> [w3857]
                                in-place-border: [w3854] -> w3846
                                n1307 = in-place-cluster #24(w3852) -> ("aAO"=w3856:u32[])
                                n1308 = call "add channel to active arrayv2.vi"("line array in"=w3856, "line to add"=w3857) -> ("line array out"=w3855:u32[], "addition"=w3854:bool)  [unwired: 1 out]
                                n1309 = in-place-cluster #24("aAO"=w3855) -> (w3850:T10)
                                }
                                n1310 = call "2pparameters.vi"("Params in"=w3850, "command"="set") -> ()  [unwired: 1 out]
                                }
                                frame #2 {
                                n1311 = call "2pparameters.vi"("command"="get") -> ("params out"=w3863:T10)  [unwired: 1 in]
                                n1312 = Unbundle By Name(w3863) -> ("autoshutter"=w3862:bool, "wavdet"=w3858:bool)
